vi "string match filter.vi"(10 "string filter value":string, 11 "string value":string) -> (3 "match?":bool)   [LabVIEW 2016, in "FPGA RM System Definition API.lvlib"]
uses:
  FPGA RM System Definition API.lvlib
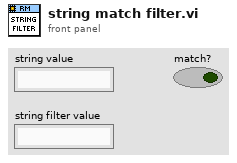
[diagram p1: front panel]
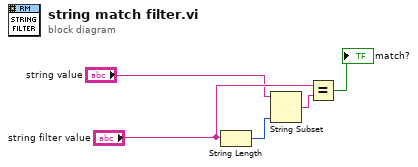
[diagram p0: block diagram]
diagram:
  n1 = String Length(string="string filter value") -> (length=w2:i32)
  n2 = String Subset(string="string value", length (rest)=w2) -> (substring=w3:string)  [unwired: 1 in]
  n3 = Equal?(x="string filter value", y=w3) -> (x = y?=→"match?":bool)
